vi "Disable if False.vi"(1 "Boolean":bool) -> (0 "Disabled State out":u8)   [LabVIEW 2013]
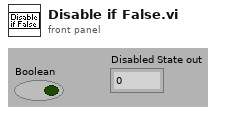
[diagram p1: front panel]
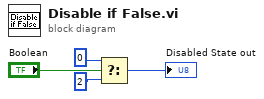
[diagram p0: block diagram]
diagram:
  n1 = Select(t=u8 0 ("Disabled"), s="Boolean", f=u8 2 ("Disabled")) -> (s? t:f=→"Disabled State out":u8)
